vi "Write MultipartData.vi"(8 "error in (no error)":errorcluster, 10 "Multipart Post data":T1[](array[typedef]), 11 "httpRequest in":refnum<class "httpRequest.lvclass">) -> (0 "error out":errorcluster, 3 "httpRequest out":refnum<class "httpRequest.lvclass">)   [LabVIEW 2020, in "httpClient.lvlib" / "httpRequest.lvclass"]
uses:
  httpRequest.lvclass
  Multipart data -- cluster.ctl
  httpRequest.lvclass/httpRequest.ctl
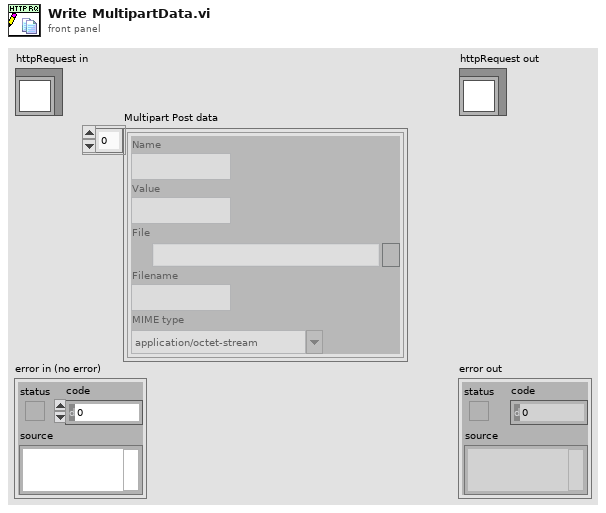
[diagram p1: front panel]
types:
  T1 = typedef "httpClient.lvlib/httpRequest.lvclass/Multipart data -- cluster.ctl" = cluster{"Name":string, "Value":string, "File":path, "Filename":string, "MIME type":string}
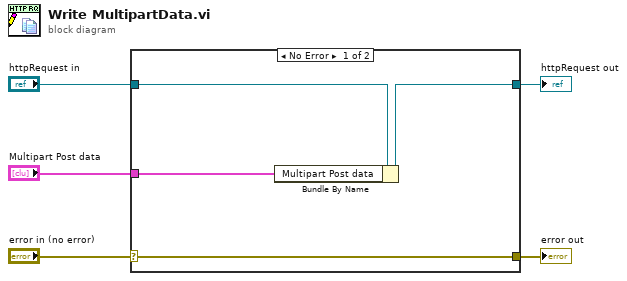
[diagram p0: block diagram]
diagram:
  n1 = case shown="No Error" "error in (no error)" {
    selector: "error in (no error)" -> [w9 w10]
    tunnel: [w9 w10] -> w4
    tunnel: [w6 w11] -> w2
    tunnel: "httpRequest in" -> [w8 w11]
    tunnel: "Multipart Post data" -> [w7 _]
    frame No Error {
      n2 = Bundle By Name(cluster=w8, "Multipart Post data"=w7) -> (w6:refnum<class "httpRequest.lvclass">)
    }
    frame Error {
    }
  }
  "error out" <- w4
  "httpRequest out" <- w2
